vi "rspvtd_Show Worker Front Panel.vi"(8 "error in":errorcluster, 11 "Data in":variant) -> (0 "error out":errorcluster, 3 "Data out":T1)   [LabVIEW 2017, in "Application Manager.lvclass"]
doc: "This VI converts variant data contained in the associated <b>Public API Response</b> message to its correct data type.\n---"
uses:
  Application Manager.lvclass
  rsp_Show Worker Front Panel.ctl
  Common VIs/DC_UID.ctl
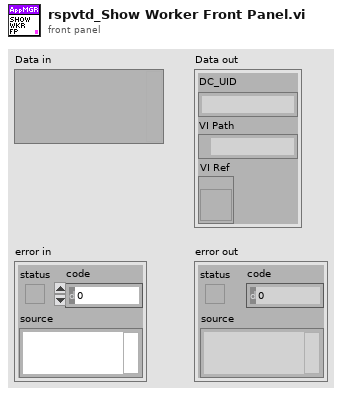
[diagram p1: front panel]
types:
  T1 = typedef "Application Manager.lvclass/rsp_Show Worker Front Panel.ctl" = cluster{"DC_UID":T2, "VI Path":path, "VI Ref":refnum<vi>}
  T2 = typedef "DC_UID.ctl" = string
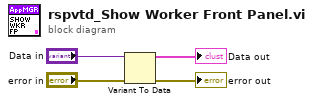
[diagram p0: block diagram]
diagram:
  n1 = Variant To Data(error in="error in", Variant="Data in") -> (data=→"Data out":T1, error out=→"error out":errorcluster)  [unwired: 1 in]
